vi "Read data (recall mode).vi"(0 "aNETka config":i32[](array[numeric])=[2, 5, 1], 4 "Data file path":path, 11 "Up Inputs":sgl[](array[numeric])=[511.0, 11.02656] format="%.2f", 13 "Down Inputs":sgl[](array[numeric])=[1.0, 20.0] format="%.2f") -> (8 "Inputs":string[](array[string])=["Input 1", "Input 2"], 12 "Continue? (T=yes)":bool=TRUE, 14 "Scaled inputs":sgl[][](array[numeric])=[[0.05, 0.05], [0.051761255, 0.13162111], [0.05528376, 0.2173232], [0.062328767, 0.30731055], [0.07641879, 0.4017972], [0.10459883, 0.5010081], [0.1609589, 0.6051796], [0.27367905, 0.7145597], [0.49911937, 0.82940876], [0.95, 0.95000035]] format="%.2f", 18 "Inputs":sgl[][](array[numeric])=[[1.0, 20.0], [2.0, 21.0], [4.0, 22.05], [8.0, 23.1525], [16.0, 24.310125], [32.0, 25.52563], [64.0, 26.801912], [128.0, 28.142008], [256.0, 29.549109], [512.0, 31.026564]] format="%.2f")   [LabVIEW 2010]
uses:
  <vilib>/Utility/file.llb/Read From Spreadsheet File (DBL).vi
panel:
  in  "OK":bool
  in  "Exit":bool
  in  "Inputs start at column \n(type number from first row below)":i32 min=0 max=1000 step=1
  out "Column nr":i32[](array[numeric])=[0, 1, 2]
  out "Column\ncaptions":string[](array[string])=["Input 1", "Input 2", "Output 1"]
  out "Data":sgl[][](array[numeric])=[[1.0, 20.0, 1.1052631], [2.0, 21.0, 1.2105263], [4.0, 22.05, 1.4432133], [8.0, 23.1525, 2.0559313], [16.0, 24.310125, 4.850724], [32.0, 25.52563, -8.885134], [64.0, 26.801912, -2.4410372], [128.0, 28.142008, -1.5636406], [256.0, 29.549109, -1.2609758], [512.0, 31.026564, -1.1290157]] step=0.05 format="%.2f"
  # "Rows\nColumns"
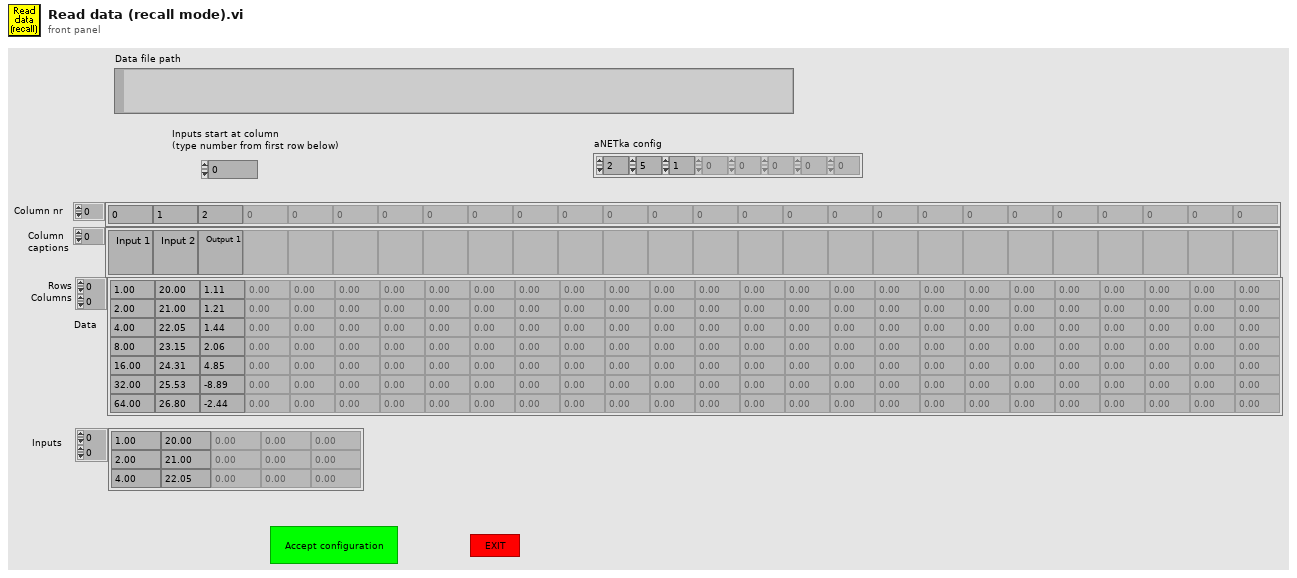
[diagram p1: front panel]
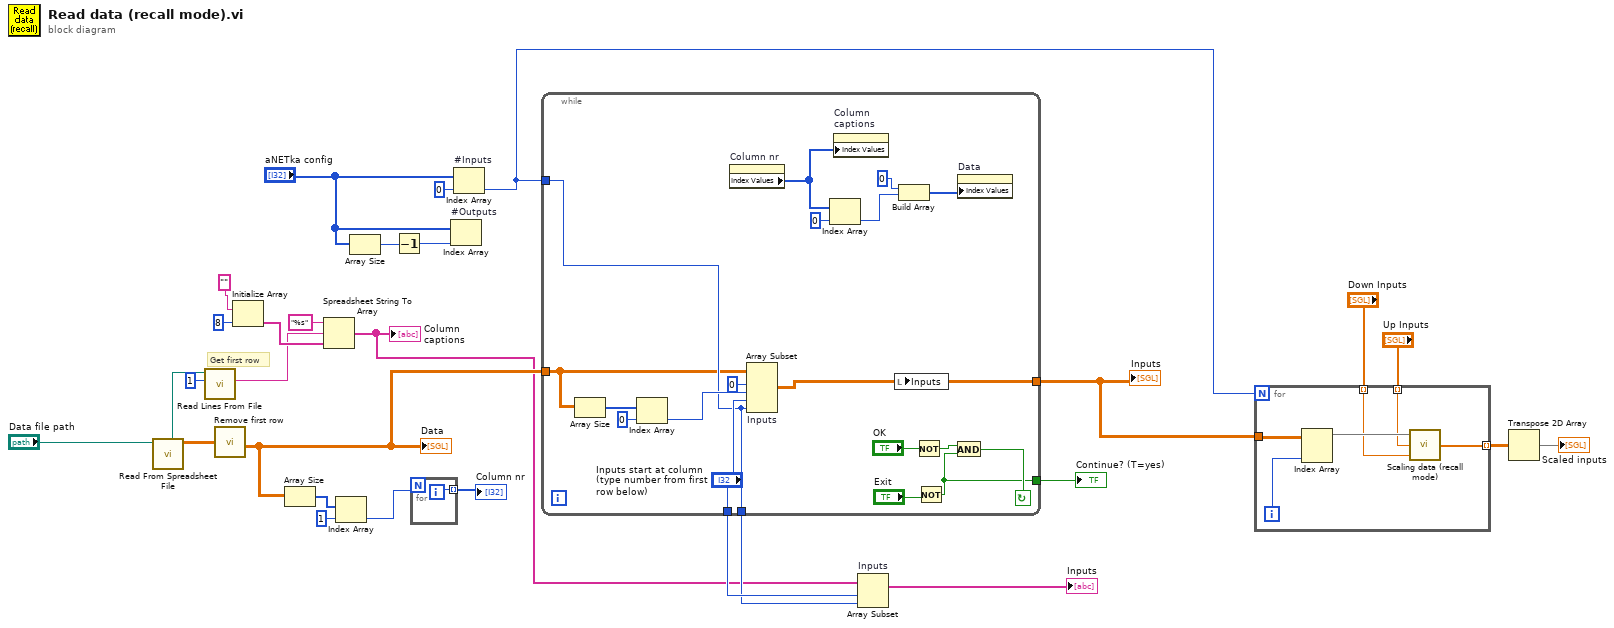
[diagram p0: block diagram]
diagram:
  # "Get first row"
  n1 = call-poly <vilib>:"Read From Spreadsheet File.vi"("file path (dialog if empty)"="Data file path") -> ("all rows"=w23:dbl[][], "new file path (Not A Path if cancelled)"=w22:path)  [unwired: 6 in, 3 out]
  n2 = call <vilib>:"Read Lines From File.vi"("file path (dialog if empty)"=w22, "number of lines (all:-1)"=1) -> ("line string"=w24:string)  [unwired: 4 in, 3 out]
  n3 = call "Remove first row.vi"("Data with comments\nin first row"=w23) -> ("The same data\nwithout first raw"=w15:sgl[][])
  "Data" <- w15
  n4 = Initialize Array("", 8 ("Dimension Size")) -> (w27:string[])
  n5 = Array Size(array=w15) -> (size(s)=w21:i32[])
  n6 = Spreadsheet String To Array(format string="%s", spreadsheet string=w24, array type (2D Dbl)=w27) -> (array=w4:string[])  [unwired: 1 in]
  "Column\ncaptions" <- w4
  n7 = Index Array(array=w21, index=1 ("Index")) -> (element=w19:i32)
  n8 = Array Size(array="aNETka config") -> (size(s)=w12:i32)
  n9 = Decrement(x=w12) -> (x-1=w11:i32)
  n10 = for {
    N: w19 -> [_]
    tunnel: [w30] -> w18 mode=indexing
    i -> [w30]
  }
  "Column nr" <- w18
  n11 = Index Array "#Outputs"(array="aNETka config", index=w11) -> ()  [unwired: 1 out]
  n12 = Index Array "#Inputs"(array="aNETka config", index=0 ("Index")) -> (element=w8:i32)
  n13 = while {
    tunnel: [w32] -> w6
    tunnel: ["Inputs start at column \n(type number from first row below)"] -> w7
    tunnel: [w34] -> w10
    tunnel: w8 -> [w32]
    tunnel: w15 -> [w31]
    tunnel: [w44] -> w16
    stop <- w45 continue-if-true
    n14 = Array Size(array=w31) -> (size(s)=w33:i32[])
    n15 = Index Array(array=w33, index=0 ("Index")) -> (element=w35:i32)
    n16 = property on="Column nr" class="Arr (strict)"() -> ("Index Values"=w42:u32[])  [unwired: 2 in, 2 out]
    n17 = Array Subset "Inputs"(array=w31, index (row)=0 ("Array Index"), length (row)=w35, index (col)="Inputs start at column \n(type number from first row below)", length (col)=w32) -> (w34:sgl[][])
    n18 = Index Array(array=w42, index=0 ("Index")) -> (element=w41:u32)
    n19 = property on="Column\ncaptions" class="Arr (strict)"("Index Values"=w42) -> ()  [unwired: 2 in, 2 out]
    n20 = local write "Inputs"(w34) -> ()
    n21 = Build Array(0, w41) -> (w43:u32[])
    n22 = Not(x="OK") -> (.not. x?=w47:bool)
    n23 = Not(x="Exit") -> (.not. x?=w44:bool)
    n24 = And(x=w47, y=w44) -> (x .and. y?=w45:bool)
    n25 = property on="Data" class="Arr (strict)"("Index Values"=w43) -> ()  [unwired: 2 in, 2 out]
  }
  "Continue? (T=yes)" <- w16
  "Inputs" <- w10
  n26 = Array Subset "Inputs"(array=w4, index=w7, length=w6) -> (→"Inputs":string[])
  n27 = for {
    N: w8 -> [_]
    tunnel: w10 -> [w53]
    tunnel: [w52] -> w1 mode=indexing
    tunnel: "Up Inputs" -> [w50] mode=indexing
    tunnel: "Down Inputs" -> [w49] mode=indexing
    i -> [w54]
    n28 = Index Array(array=w53, index (col)=w54) -> (element=w51:sgl[])  [unwired: 1 in]
    n29 = call "Scaling data (recall mode).vi"("Offset down"=w49, "Offset up"=w50, "Input data"=w51) -> ("Scaled data"=w52:sgl[])
  }
  n30 = Transpose 2D Array(2D array=w1) -> (transposed array=→"Scaled inputs":sgl[][])
